vi "Calculate Rotation Matrix.vi"(1 "data AGM - XYZ":dbl[](array[numeric])) -> (0 "Rotation Matrix":T1)   [LabVIEW 2021, in "IMU Processing.lvlib"]
uses:
  IMU Processing.lvlib
  <vilib>/Analysis/Matrix/Datatypes/RealMatrix.ctl
  <vilib>/Analysis/_algsub.llb/Real Vector Norm.vi
  <vilib>/Analysis/NI_AALPro.lvlib
  <vilib>/Analysis/Matrix/NI_Matrix.lvlib
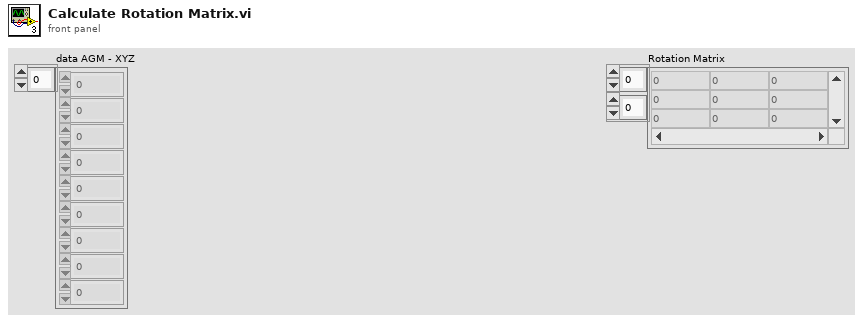
[diagram p1: front panel]
types:
  T1 = typedef "NI_Matrix.lvlib/RealMatrix.ctl" = dbl[][]
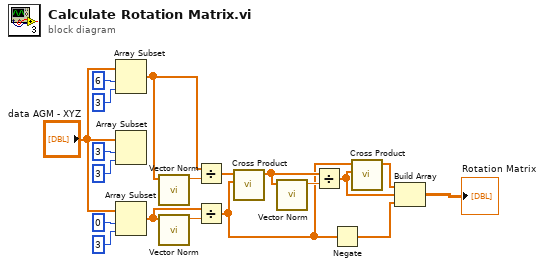
[diagram p0: block diagram]
diagram:
  n1 = Array Subset(array="data AGM - XYZ", index=6, length=3) -> (w7:dbl[])
  n2 = Array Subset(array="data AGM - XYZ", index=3, length=3) -> ()  [unwired: 1 out]
  n3 = Array Subset(array="data AGM - XYZ", index=0, length=3) -> (w9:dbl[])
  n4 = call-poly <vilib>:"Vector Norm.vi"("Input Vector"=w7) -> ("norm"=w11:dbl)  [unwired: 9 in, 1 out]
  n5 = call-poly <vilib>:"Vector Norm.vi"("Input Vector"=w9) -> ("norm"=w12:dbl)  [unwired: 9 in, 1 out]
  n6 = Divide(x=w7, y=w11) -> (x/y=w6:dbl[])
  n7 = Divide(x=w9, y=w12) -> (x/y=w2:dbl[])
  n8 = call <vilib>:"Cross Product.vi"("B Vector"=w2, "A Vector"=w6) -> ("Cross Product"=w8:dbl[])  [unwired: 8 in, 1 out]
  n9 = call-poly <vilib>:"Vector Norm.vi"("Input Vector"=w8) -> ("norm"=w10:dbl)  [unwired: 9 in, 1 out]
  n10 = Divide(x=w8, y=w10) -> (x/y=w4:dbl[])
  n11 = Negate(x=w2) -> (-x=w1:dbl[])
  n12 = call <vilib>:"Cross Product.vi"("B Vector"=w4, "A Vector"=w2) -> ("Cross Product"=w5:dbl[])  [unwired: 8 in, 1 out]
  n13 = Build Array(w5, w4, w1) -> (→"Rotation Matrix":T1)
